vi "WhetherInnerOrOn.vi"(1 "Error permitted":dbl, 2 "JudgePoint":dbl[](array[numeric]), 3 "InputPolygon":dbl[][](array[numeric])) -> (0 "Point on or inside?":bool)   [LabVIEW 2013]
panel:
  out "Numeric":i32
  out "arccos(x)":dbl
  out "x+y":dbl
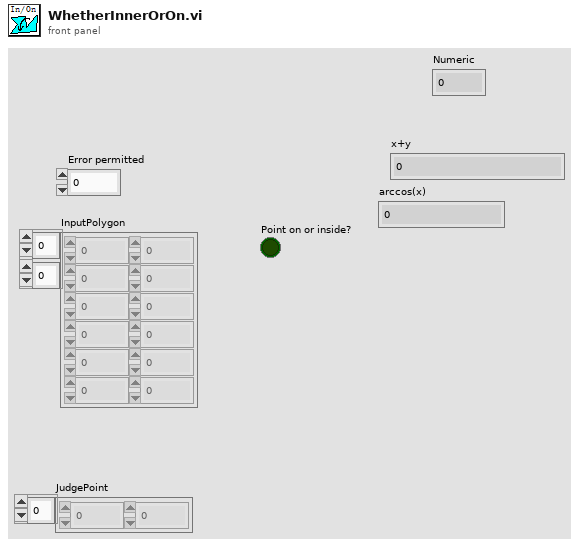
[diagram p1: front panel]
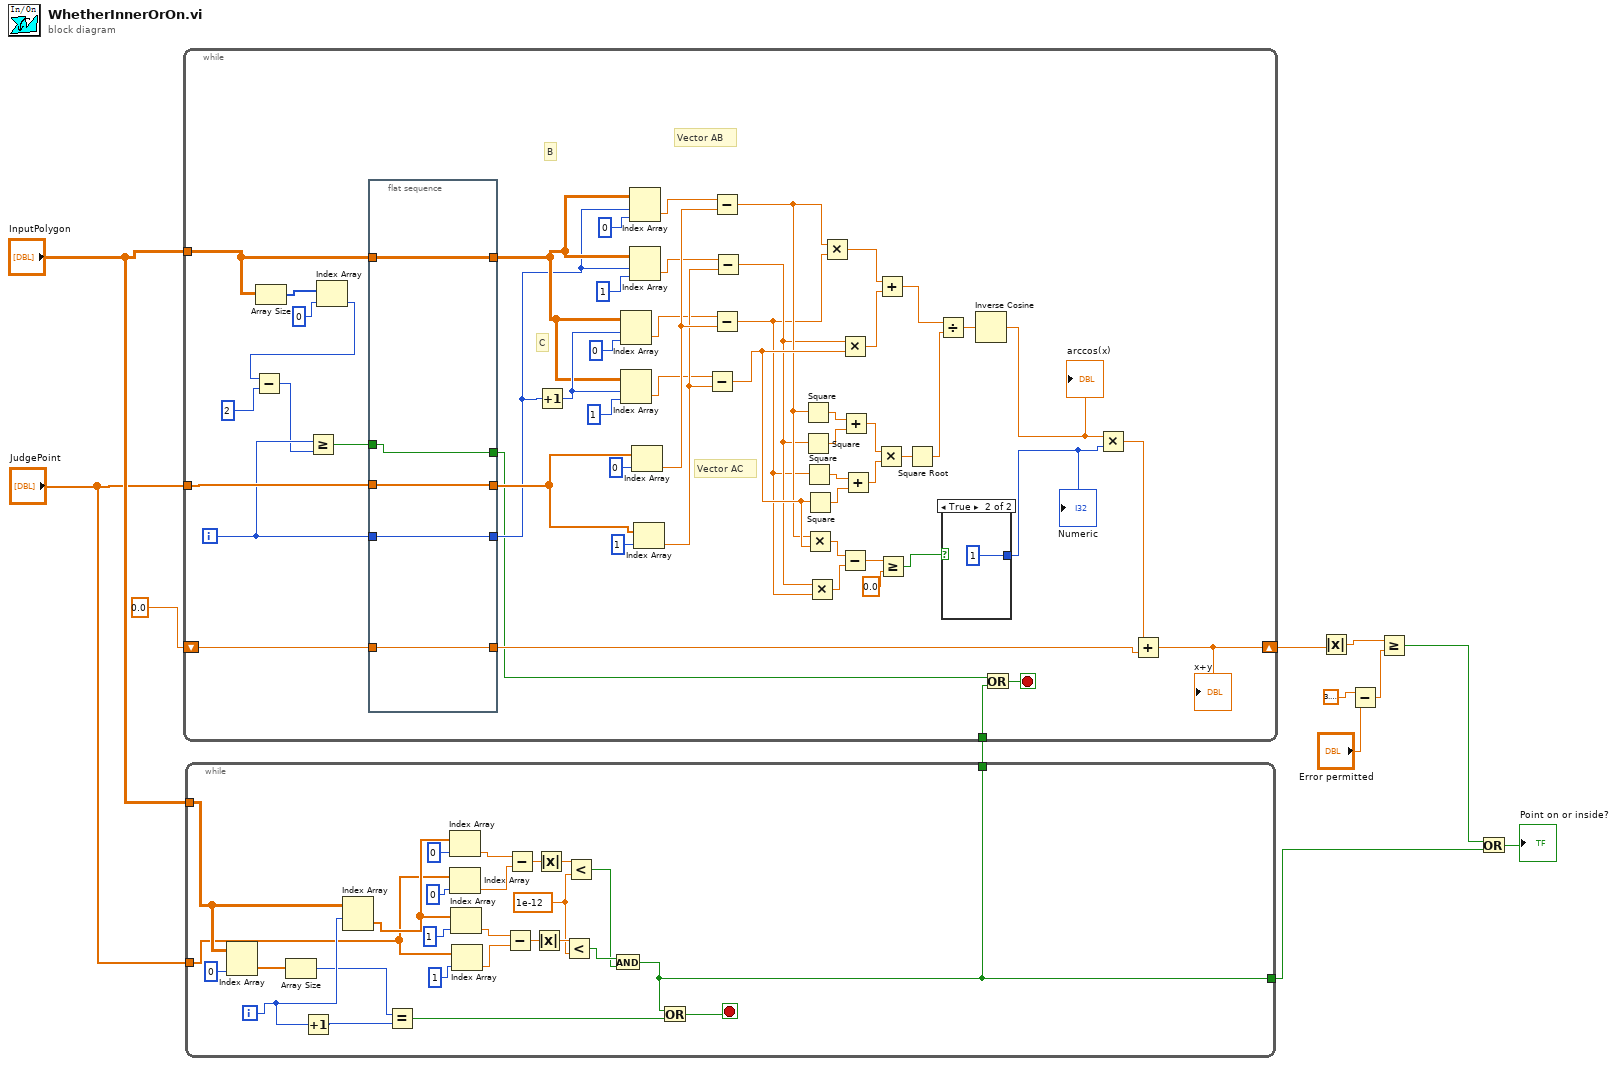
[diagram p0: block diagram]
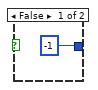
[diagram p2: hidden frame]
diagram:
  n1 = while {
    tunnel: "InputPolygon" -> [w38]
    tunnel: "JudgePoint" -> [w29]
    tunnel: [w13] -> w2
    tunnel: [w13] -> w1
    i -> [w34]
    stop <- w31 stop-if-true
    w16 = 1e-12
    n2 = Index Array(array=w38, index (col)=0 ("disabled index (col)")) -> (element=w36:dbl[])  [unwired: 1 in]
    n3 = Array Size(array=w36) -> (size(s)=w33:i32)
    n4 = Increment(x=w34) -> (x+1=w35:i32)
    n5 = Index Array(array=w38, index (row)=w34) -> (element=w30:dbl[])  [unwired: 1 in]
    n6 = Equal?(x=w33, y=w35) -> (x = y?=w32:bool)
    n7 = Index Array(array=w30, index=0) -> (element=w24:dbl)
    n8 = Index Array(array=w29, index=0) -> (element=w23:dbl)
    n9 = Index Array(array=w30, index=1) -> (element=w18:dbl)
    n10 = Index Array(array=w29, index=1) -> (element=w17:dbl)
    n11 = Subtract(x=w18, y=w17) -> (x-y=w20:dbl)
    n12 = Subtract(x=w24, y=w23) -> (x-y=w22:dbl)
    n13 = Absolute Value(x=w20) -> (abs(x)=w19:dbl)
    n14 = Absolute Value(x=w22) -> (abs(x)=w21:dbl)
    n15 = Less?(x=w19, y=w16) -> (x < y?=w15:bool)
    n16 = Less?(x=w21, y=w16) -> (x < y?=w14:bool)
    n17 = And(x=w15, y=w14) -> (x .and. y?=w13:bool)
    n18 = Or(x=w13, y=w32) -> (x .or. y?=w31:bool)
  }
  n19 = while {
    tunnel: "InputPolygon" -> [w58]
    tunnel: "JudgePoint" -> [w54]
    shift-right: [w60] -> w8
    shift-left: 0.0 -> [w56]
    tunnel: w1 -> [w39]
    i -> [w52]
    stop <- w41 stop-if-true
    # "Vector AC"
    # "C"
    # "B"
    # "Vector AB"
    n20 = Array Size(array=w58) -> (size(s)=w93:i32[])
    n21 = Index Array(array=w93, index=0) -> (element=w44:i32)
    n22 = Subtract(x=w44, y=2 ("index")) -> (x-y=w43:i32)
    n23 = Greater Or Equal?(x=w52, y=w43) -> (x >= y?=w59:bool)
    n24 = flat-sequence {
      tunnel: w59 -> [w100]
      tunnel: [w100] -> w40
      tunnel: w58 -> [w99]
      tunnel: [w99] -> w57
      tunnel: w56 -> [w98]
      tunnel: [w98] -> w55
      tunnel: [w97] -> w53
      tunnel: w54 -> [w97]
      tunnel: w52 -> [w96]
      tunnel: [w96] -> w51
      frame #0 {
      }
    }
    n25 = Increment(x=w51) -> (x+1=w85:i32)
    n26 = Index Array(array=w57, index (row)=w85, index (col)=0 ("disabled index (col)")) -> (element=w81:dbl)
    n27 = Index Array(array=w57, index (row)=w85, index (col)=1 ("disabled index (col)")) -> (element=w79:dbl)
    n28 = Index Array(array=w57, index (row)=w51, index (col)=0 ("disabled index (col)")) -> (element=w82:dbl)
    n29 = Index Array(array=w57, index (row)=w51, index (col)=1 ("disabled index (col)")) -> (element=w80:dbl)
    n30 = Index Array(array=w53, index=0) -> (element=w84:dbl)
    n31 = Index Array(array=w53, index=1) -> (element=w83:dbl)
    n32 = Subtract(x=w79, y=w83) -> (x-y=w66:dbl)
    n33 = Subtract(x=w82, y=w84) -> (x-y=w65:dbl)
    n34 = Subtract(x=w81, y=w84) -> (x-y=w63:dbl)
    n35 = Subtract(x=w80, y=w83) -> (x-y=w64:dbl)
    n36 = Square(x=w65) -> (x^2=w76:dbl)
    n37 = Square(x=w64) -> (x^2=w75:dbl)
    n38 = Square(x=w63) -> (x^2=w74:dbl)
    n39 = Square(x=w66) -> (x^2=w73:dbl)
    n40 = Multiply(x=w65, y=w66) -> (x*y=w62:dbl)
    n41 = Multiply(x=w64, y=w63) -> (x*y=w61:dbl)
    n42 = Multiply(x=w65, y=w63) -> (x*y=w78:dbl)
    n43 = Multiply(x=w64, y=w66) -> (x*y=w77:dbl)
    n44 = Subtract(x=w62, y=w61) -> (x-y=w48:dbl)
    n45 = Add(x=w76, y=w75) -> (x+y=w71:dbl)
    n46 = Add(x=w74, y=w73) -> (x+y=w72:dbl)
    n47 = Multiply(x=w71, y=w72) -> (x*y=w70:dbl)
    n48 = Add(x=w78, y=w77) -> (x+y=w69:dbl)
    n49 = Greater Or Equal?(x=w48, y=0.0) -> (x >= y?=w46:bool)
    n50 = Square Root(x=w70) -> (sqrt(x)=w68:dbl)
    n51 = Divide(x=w69, y=w68) -> (x/y=w67:dbl)
    n52 = case shown="True" w46 {
      tunnel: [-1 1] -> w45
      frame False {
      }
      frame True {
      }
    }
    "Numeric" <- w45
    n53 = Inverse Cosine(1:w67) -> (0:w49:dbl)
    "arccos(x)" <- w49
    n54 = Or(x=w40, y=w39) -> (x .or. y?=w41:bool)
    n55 = Multiply(x=w49, y=w45) -> (x*y=w50:dbl)
    n56 = Add(x=w50, y=w55) -> (x+y=w60:dbl)
    "x+y" <- w60
  }
  n57 = Absolute Value(x=w8) -> (abs(x)=w7:dbl)
  n58 = Subtract(x=3.141592653589793, y="Error permitted") -> (x-y=w11:dbl)
  n59 = Greater Or Equal?(x=w7, y=w11) -> (x >= y?=w6:bool)
  n60 = Or(x=w6, y=w2) -> (x .or. y?=→"Point on or inside?":bool)
